vi "dfd_Bilinear Prewarping.vi"(1 "w":dbl format="%.2f") -> (0 "prewarped w":dbl format="%.2f")   [LabVIEW 2017, in "NI_DigFilter_Design.lvlib"]
uses:
  <vilib>/addons/Digital Filter Design/NI_DigFilter_Design.lvlib
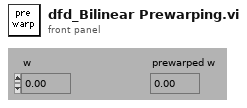
[diagram p1: front panel]
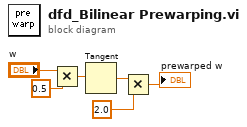
[diagram p0: block diagram]
diagram:
  n1 = Multiply(x="w", y=0.5) -> (x*y=w1:dbl)
  n2 = Tangent(1:w1) -> (0:w4:dbl)
  n3 = Multiply(x=w4, y=2.0) -> (x*y=→"prewarped w":dbl)
